vi "Remote Client.vi"(6 "Wait for Response?":bool, 8 "error in (no error)":errorcluster, 9 "Data":variant, 10 "Command":string, 11 "Instrument in":refnum<class "Instrument.lvclass">) -> (0 "error out":errorcluster, 1 "Data out":variant, 2 "Command out":string, 3 "Instrument out":refnum<class "Instrument.lvclass">)   [LabVIEW 2016, in "Instrument.lvclass"]
uses:
  Instrument.lvclass
  Instrument.lvclass/Instrument.ctl
  RemoteControl/RemoteControl.lvclass
  RemoteControl.STM/RemoteControl.STM.lvclass
  C:/user/patrick/hg/levylab_inst/lvsrc/SMOs/RemoteControl/RemoteControl.lvclass
  <userlib>/_OpenG.lib/numeric/numeric.llb/Random Number Within Range - I32__ogtk.vi
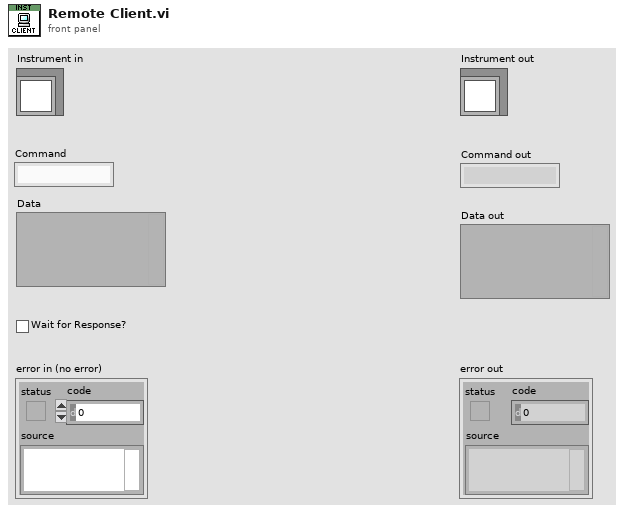
[diagram p1: front panel]
types:
  T1 = typedef "Instrument.lvclass/PublicEvents--Cluster.ctl" = cluster{"MessageFromProcess":refnum<user-event>}
  T2 = typedef "Instrument.lvclass/SMO RC Type--enum.ctl" = enum16{"RC", "STM", "ZMQ"}
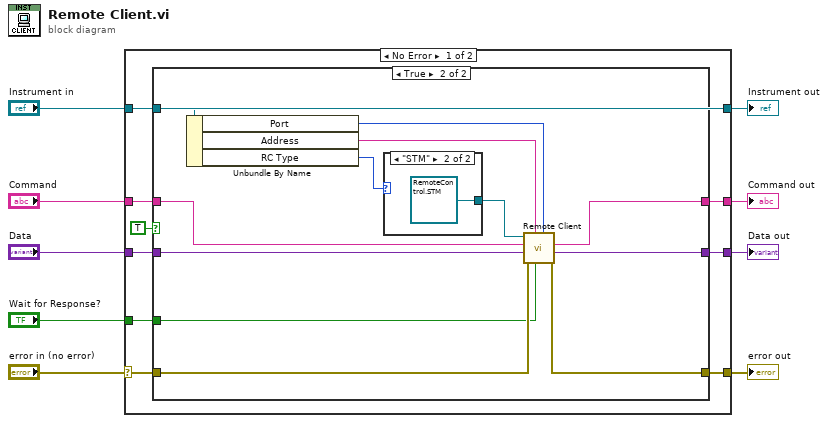
[diagram p0: block diagram]
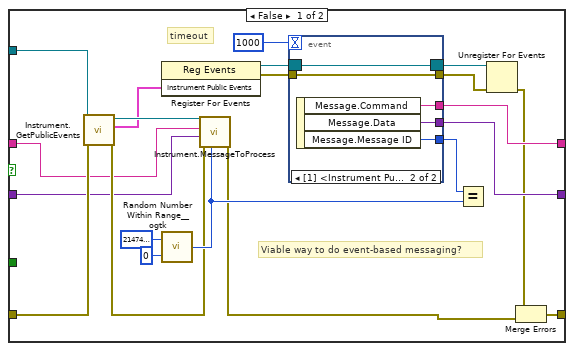
[diagram p2: hidden frame]
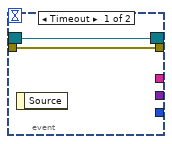
[diagram p3: hidden frame]
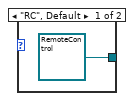
[diagram p4: hidden frame]
diagram:
  n1 = case shown="No Error" "error in (no error)" {
    selector: "error in (no error)" -> [w18 w62]
    tunnel: [w17 w62] -> w8
    tunnel: [w13 w61] -> w6
    tunnel: "Instrument in" -> [w13 w61]
    tunnel: [w16 _] -> w5
    tunnel: [w11 _] -> w4
    tunnel: "Command" -> [w12 _]
    tunnel: "Data" -> [w15 _]
    tunnel: "Wait for Response?" -> [w14 _]
    frame No Error {
      n2 = case shown="True" TRUE {
        tunnel: w18 -> [w27 w58]
        tunnel: [w20 w57] -> w17
        tunnel: [w33 w56] -> w16
        tunnel: w15 -> [w25 w55]
        tunnel: w14 -> [_ w54]
        tunnel: w13 -> [w37 w49]
        tunnel: w12 -> [w24 w48]
        tunnel: [w23 w47] -> w11
        frame False {
          # "Viable way to do event-based messaging?"
          # "timeout"
          n3 = call "Instrument.GetPublicEvents.vi"("error in (no error)"=w27, "Instrument"=w37) -> ("error out"=w26:errorcluster, "Instrument Public Events"=w35:T1, "Instrument out"=w36:refnum<class "Instrument.lvclass">)  [unwired: 7 in]
          n4 = register-events(w35) -> (reference out=w34:refnum<event-registration>, error out=w30:errorcluster)  [unwired: 2 in]
          n5 = call-poly <userlib>:"Random Number Within Range__ogtk.vi"("High"=2147483647, "Low"=0) -> ("Random Number"=w29:i32)  [unwired: 3 in]
          n6 = call "Instrument.MessageToProcess.vi"("Message ID"=w29, "error in (no error)"=w26, "Message.Data"=w25, "Message.Command"=w24, "Instrument"=w36) -> ("error out"=w19:errorcluster)  [unwired: 5 in, 1 out]
          n7 = event shown="[1] <Instrument Public Events.MessageFromProcess>: User Event" {
            selector: w34 -> [w40 w42]
            dyn-events: [w40 w42] -> w22
            timeout: 1000 -> [_ _]
            tunnel: [_ w46] -> w23
            tunnel: [_ w45] -> w33
            tunnel: [w41 w44] -> w31
            tunnel: w30 -> [w41 w44]
            tunnel: [_ w43] -> w28
            event Timeout {
              n8 = event-data() -> ()  [unwired: 1 in, 1 out]
            }
            event User Event {
              n9 = event-data() -> ("Message.Command"=w46:string, "Message.Data"=w45:variant, "Message.Message ID"=w43:i32)  [unwired: 1 in]
            }
          }
          n10 = Equal?(x=w28, y=w29) -> ()  [unwired: 1 out]
          n11 = Unregister For Events(event registration refnum=w22, error in=w31) -> (error out=w21:errorcluster)
          n12 = Merge Errors(w21, w19) -> (w20:errorcluster)
        }
        frame True {
          n13 = Unbundle By Name(w49) -> ("Port"=w53:u16, "Address"=w52:string, "RC Type"=w51:T2)
          n14 = case shown="\"STM\"" w51 {
            tunnel: [refnum<class "RemoteControl.lvclass"> refnum ("RemoteControl in") refnum<class "RemoteControl.STM.lvclass"> refnum ("RemoteControl.STM.lvclass")] -> w50
            frame "RC", Default {
            }
            frame "STM" {
            }
          }
          n15 = call "Remote Client.vi"("Port"=w53, "Wait for Response?"=w54, "address"=w52, "error in (no error)"=w58, "Data"=w55, "Command"=w48, "RemoteControl in"=w50) -> ("error out"=w57:errorcluster, "Data out"=w56:variant, "Command out"=w47:string)  [unwired: 1 in, 1 out]
        }
      }
    }
    frame Error {
    }
  }
  "error out" <- w8
  "Instrument out" <- w6
  "Command out" <- w4
  "Data out" <- w5
